vi "Log File.vi"(8 "error in":errorcluster, 9 "Test Result":T1, 11 "Sequence Context":refnum<k7>) -> (0 "error out":errorcluster)   [LabVIEW 2021, in "OPC UA.lvlib" / "PostUUT.lvclass"]
uses:
  PostUUT.lvclass
  <vilib>/addons/TestStand/_TSUtility.llb/TestStand - Get Property Value (String).vi
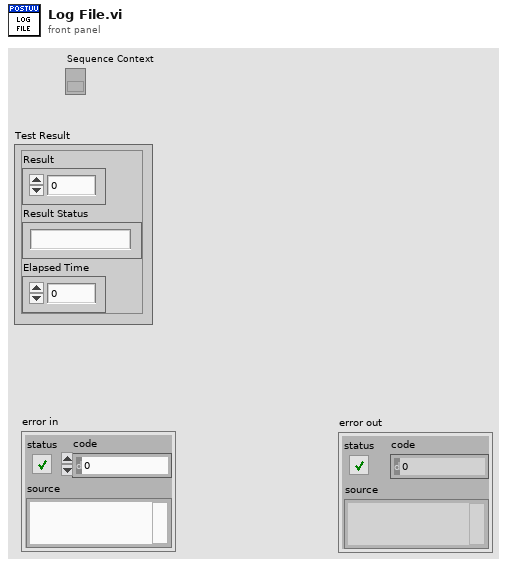
[diagram p1: front panel]
types:
  T1 = cluster{"Result":i32, "Result Status":string, "Elapsed Time":i32}
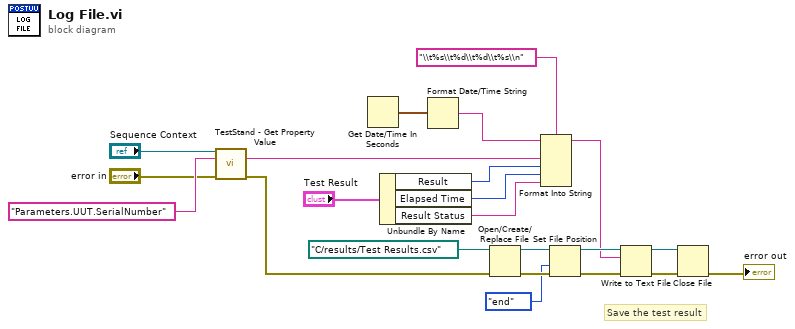
[diagram p0: block diagram]
diagram:
  # "Save the test result"
  n1 = call-poly <vilib>:"TestStand - Get Property Value.vi"("Sequence Context In"="Sequence Context", "Lookup String"="Parameters.UUT.SerialNumber", "error in (no error)"="error in") -> ("Value"=w5:string, "error out"=w7:errorcluster)  [unwired: 10 in, 1 out]
  n2 = Get Date/Time In Seconds() -> (seconds since 1Jan1904=w11:timestamp)
  n3 = Unbundle By Name("Test Result") -> ("Result"=w3:i32, "Elapsed Time"=w2:i32, "Result Status"=w1:string)
  n4 = Format Date/Time String(seconds (now)=w11) -> (date/time string=w10:string)  [unwired: 2 in]
  n5 = Open/Create/Replace File(file path (use dialog)=path "C:/results/Test Results.csv" ("file path"), error in=w7) -> (refnum out=w20:refnum<file>, error out=w18:errorcluster)  [unwired: 4 in, 1 out]
  n6 = Format Into String(format string="\\t%s\\t%d\\t%d\\t%s\\n", initial string=w10, w5, w3, w2, w1) -> (resulting string=w13:string)  [unwired: 1 in, 1 out]
  n7 = Set File Position(refnum=w20, from (0:start)=enum16{"start", "end", "current"}."end", error in=w18) -> (refnum out=w19:refnum<file>, error out=w17:errorcluster)  [unwired: 1 in]
  n8 = Write to Text File(file (use dialog)=w19, text=w13, error in=w17) -> (refnum out=w21:refnum<file>, error out=w22:errorcluster)  [unwired: 1 in, 1 out]
  n9 = Close File(refnum=w21, error in=w22) -> (error out=→"error out":errorcluster)  [unwired: 1 out]
